vi "dsdll_initialize.vi"(8 "error in":errorcluster, 11 "path to dsdll.dll (optional)":path) -> (0 "error out":errorcluster, 3 "dsdll instance out":T1)   [LabVIEW 2020, in "dsdll.lvlib"]
doc: "Call this before using any other function in DSDLL.\n\nIf no 'dsdll.dll' path is specified, the DSDLL library expects 'dsdll.dll' in application root directory i.e. the same as top level of the LV project or the folder with the compiled application executable."
uses:
  dsdll.lvlib
  dsdll_instance.ctl
  dsdll_device_record.ctl
  <vilib>/Utility/error.llb/Error Cluster From Error Code.vi
  <vilib>/ErrorRing/Error Ring.xnode
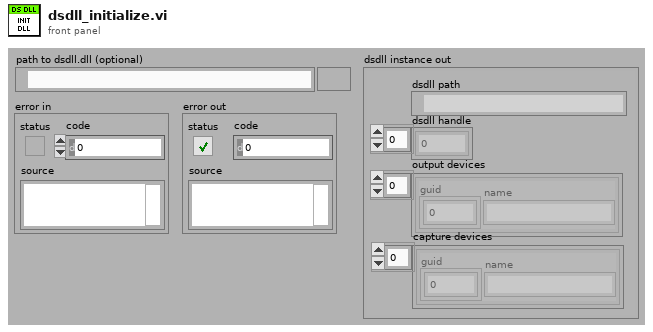
[diagram p1: front panel]
types:
  T1 = typedef "dsdll.lvlib/dsdll_instance.ctl" = cluster{"dsdll path":path, "dsdll handle":u8[], "output devices":T2[], "capture devices":T2[]}
  T2 = typedef "dsdll.lvlib/dsdll_device_record.ctl" = cluster{"guid":u8[], "name":string}
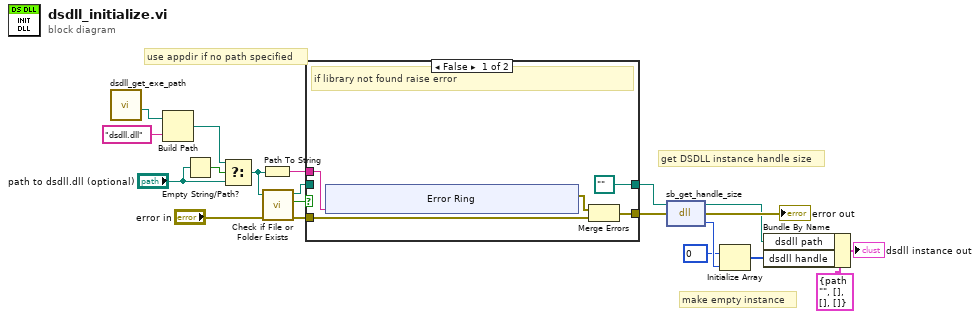
[diagram p0: block diagram]
diagram:
  # "make empty instance"
  # "get DSDLL instance handle size"
  # "use appdir if no path specified"
  n1 = call "dsdll_get_exe_path.vi"() -> ("directory path"=w1:path)  [unwired: 3 out]
  n2 = Build Path(base path=w1, name or relative path="dsdll.dll") -> (appended path=w20:path)
  n3 = Empty String/Path?(string/path="path to dsdll.dll (optional)") -> (empty?=w18:bool)
  n4 = Select(t=w20, s=w18, f="path to dsdll.dll (optional)") -> (s? t:f=w15:path)
  n5 = Path To String(path=w15) -> (string=w16:string)
  n6 = call <vilib>:"Check if File or Folder Exists.vi"("error in (no error)"="error in", "path"=w15) -> ("error out"=w13:errorcluster, "file or folder exists?"=w14:bool, "dup path"=w12:path)  [unwired: 7 in]
  n7 = case shown="False" w14 {
    tunnel: w16 -> [w25 _]
    tunnel: w13 -> [w23 w34]
    tunnel: [w22 w34] -> w10
    tunnel: [path "" ("dup path") w33] -> w9
    tunnel: w12 -> [_ w33]
    frame False {
      # "if library not found raise error"
      n8 = xnode "Error Ring"("parameter 0"=w25) -> ("error out"=w24:errorcluster)
      n9 = Merge Errors(w24, w23) -> (w22:errorcluster)
    }
    frame True {
    }
  }
  n10 = dll-call lib="dsdll.dll" fn="sb_get_handle_size" ("sb_get_handle_size()")(path in=w9, error in=w10) -> (path out=w2:path, error out=→"error out":errorcluster, "size [B]"=w6:u32)  [unwired: 1 in]
  n11 = Initialize Array(u8 0, w6) -> (w4:u8[])
  n12 = Bundle By Name(cluster=T1 {"dsdll path"=path "", "dsdll handle"=[], "output devices"=[], "capture devices"=[]} ("dsdll instance out"), "dsdll path"=w2, "dsdll handle"=w4) -> (→"dsdll instance out":T1)
